vi "PH_ImageCoG_Plotter.Show Data.vi"(0 "i ref in":refnum<vi>, 5 "error in":errorcluster) -> (14 "i ref out":refnum<vi>, 19 "error out":errorcluster)   [LabVIEW 2014, in "PH_ImageCoG_Plotter.lvlib"]
doc: "This VI plots the data at the GUI elements."
uses:
  PH_ImageCoG_Plotter.lvlib
  <vilib>/Analysis/NI_AALBase.lvlib
  <vilib>/Analysis/NI_AALPro.lvlib
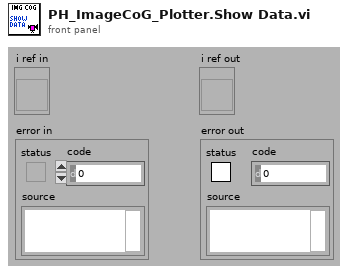
[diagram p1: front panel]
types:
  T1 = typedef "PH_ImageCoG_Plotter.lvlib/PH_ImageCoG_Plotter.i attribute.ctl" = cluster{"GUI Refs":cluster{"Delete":refnum<vi>, "Calibration status":refnum<vi>, "BI subtracted":refnum<vi>, "calc Beam Anal":refnum<vi>, "CoG - x":refnum<vi>, "CoG - y":refnum<vi>, "Type":refnum<vi>, "Center":refnum<vi>, "exp - X":refnum<vi>, "exp - Y":refnum<vi>, "Delta - X":refnum<vi>, "Delta - Y":refnum<vi>, "Available Cams":refnum<vi>, "CoG X":refnum<vi>, "CoG Y":refnum<vi>, "Delta X":refnum<vi>, "Delta Y":refnum<vi>, "Export Data":refnum<vi>, "Calibration data":refnum<vi>}, "Calibration":cluster{"Status":T2, "Calibration data":T3, "Calibration Data File":path}, "Beam Analysis":cluster{"on":bool, "exp - X":i32, "exp - Y":i32, "Type":bool, "Data":cluster{"current time":timestamp, "CoG-x":dbl, "CoG-y":dbl, "Delta-x":dbl, "Delta-y":dbl}[], "Datasets strored":i32, "Dataarray Size":i32}, "Cam instances":string[], "DIM Service Events":T4[], "Images":cluster{"Background":T7, "OP":T7, "GUI":T7}}
  T2 = typedef "PH_StatusHandler.lvlib/PH_StatusHandler.Status.ctl" = i16
  T3 = typedef "PH_ImageCalibrator.lvlib/PH_ImageCalibrator.Calibration Data.ctl" = cluster{"Date":string, "Time":string, "Cam Settings":cluster{"Cam ID":string, "Gain":dbl, "Brightness":dbl, "Shutter":dbl, "Cam Error":bool, "Mode":i32}, "Background Image":cluster{"Image":dbl[][], "Image Error":bool}, "Linear Calibration":cluster{"Calibration Factor":dbl, "not mm or mrad":bool}, "Energy Calibration":cluster{"Calibration Factor":dbl, "no mJ":bool}}
  T4 = typedef "BaseProcess.lvlib/BaseProcess.event definition.ctl" = cluster{"CAEEvtDef":T5, "Data Descriptor":T6}
  T5 = typedef "CAEObj.lvlib/CAEObj.event definition.ctl" = cluster{"URL":string, "enable":bool, "ignoreResID":bool}
  T6 = typedef "BaseProcess.lvlib/BaseProcess.descriptor string definition.ctl" = string
  T7 = typedef "IMAQ Image.ctl" = refnum<image>
  T8 = cluster{"current time":timestamp, "CoG-x":dbl, "CoG-y":dbl, "Delta-x":dbl, "Delta-y":dbl}[]
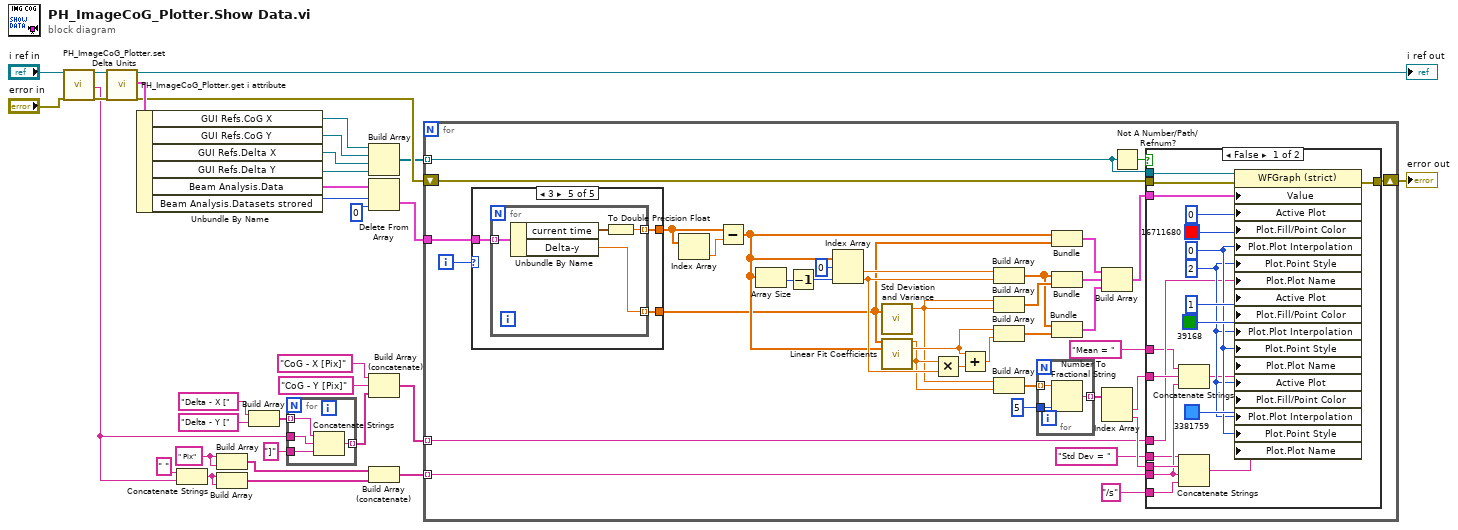
[diagram p0: block diagram]
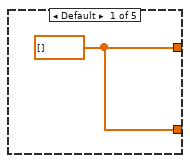
[diagram p2: hidden frame]
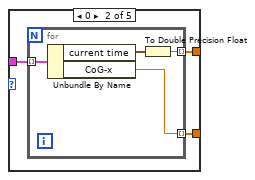
[diagram p3: hidden frame]
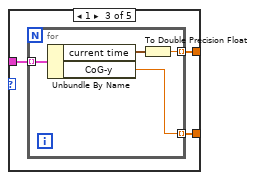
[diagram p4: hidden frame]
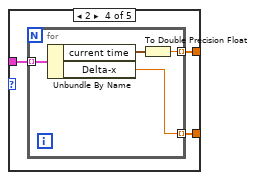
[diagram p5: hidden frame]
diagram:
  w12 = " Pix" ("Plot.Plot Name")
  n1 = call "PH_ImageCoG_Plotter.set Delta Units.vi"("i ref in"="i ref in", "error in (no error)"="error in") -> ("i ref out"=w24:refnum<vi>, "Unit"=w5:string, "error out"=w22:errorcluster)  [unwired: 15 in]
  n2 = call "PH_ImageCoG_Plotter.get i attribute.vi"("i ref in"=w24, "error in (no error)"=w22) -> ("i ref out"=→"i ref out":refnum<vi>, "i attribute"=w32:T1, "error out"=w27:errorcluster)  [unwired: 15 in]
  n3 = Unbundle By Name(w32) -> ("GUI Refs.CoG X"=w9:refnum<vi>, "GUI Refs.CoG Y"=w17:refnum<vi>, "GUI Refs.Delta X"=w16:refnum<vi>, "GUI Refs.Delta Y"=w15:refnum<vi>, "Beam Analysis.Data"=w4:T8, "Beam Analysis.Datasets strored"=w3:i32)
  n4 = Concatenate Strings(" " ("string"), w5) -> (w7:string)
  n5 = Build Array(w12, w12) -> (w13:string[])
  n6 = Build Array(w7, w7) -> (w14:string[])
  n7 = Build Array("Delta - X [" ("Plot.Plot Name"), "Delta - Y [" ("Plot.Plot Name")) -> (w18:string[])
  n8 = for {
    tunnel: w18 -> [w36] mode=indexing
    tunnel: "]" ("Plot.Plot Name") -> [w35]
    tunnel: w5 -> [w34]
    tunnel: [w33] -> w21 mode=indexing
    n9 = Concatenate Strings(w36, w34, w35) -> (w33:string)
  }
  n10 = Build Array(w9, w17, w16, w15) -> (w8:refnum<vi>[])
  n11 = Delete From Array(array=w4, length=w3, index=0) -> (deleted portion=w1:T8)  [unwired: 1 out]
  n12 = Build Array (concatenate)("CoG - X [Pix]" ("Plot.Plot Name"), "CoG - Y [Pix]" ("Plot.Plot Name"), w21) -> (w10:string[])
  n13 = Build Array (concatenate)(w13, w14) -> (w11:string[])
  n14 = for {
    tunnel: w8 -> [w70] mode=indexing
    tunnel: w11 -> [w69] mode=indexing
    shift-right: [w73] -> w31
    shift-left: w27 -> [w71]
    tunnel: w10 -> [w46] mode=indexing
    tunnel: w1 -> [w40]
    i -> [w37]
    n15 = case shown="3" w37 {
      tunnel: [w74 w77 w84 w91 w98] -> w41
      tunnel: w40 -> [_ w76 w83 w90 w97]
      tunnel: [w74 w75 w82 w89 w96] -> w38
      frame Default {
        w74 = dbl[] []
      }
      frame 0 {
        n16 = for {
          tunnel: w76 -> [w81] mode=indexing
          tunnel: [w78] -> w77 mode=indexing
          tunnel: [w80] -> w75 mode=indexing
          n17 = Unbundle By Name(w81) -> ("current time"=w79:timestamp, "CoG-x"=w80:dbl)
          n18 = To Double Precision Float(number=w79) -> (double precision float=w78:dbl)
        }
      }
      frame 1 {
        n19 = for {
          tunnel: w83 -> [w88] mode=indexing
          tunnel: [w85] -> w84 mode=indexing
          tunnel: [w87] -> w82 mode=indexing
          n20 = Unbundle By Name(w88) -> ("current time"=w86:timestamp, "CoG-y"=w87:dbl)
          n21 = To Double Precision Float(number=w86) -> (double precision float=w85:dbl)
        }
      }
      frame 2 {
        n22 = for {
          tunnel: w90 -> [w95] mode=indexing
          tunnel: [w92] -> w91 mode=indexing
          tunnel: [w94] -> w89 mode=indexing
          n23 = Unbundle By Name(w95) -> ("current time"=w93:timestamp, "Delta-x"=w94:dbl)
          n24 = To Double Precision Float(number=w93) -> (double precision float=w92:dbl)
        }
      }
      frame 3 {
        n25 = for {
          tunnel: w97 -> [w102] mode=indexing
          tunnel: [w99] -> w98 mode=indexing
          tunnel: [w101] -> w96 mode=indexing
          n26 = Unbundle By Name(w102) -> ("current time"=w100:timestamp, "Delta-y"=w101:dbl)
          n27 = To Double Precision Float(number=w100) -> (double precision float=w99:dbl)
        }
      }
    }
    n28 = Index Array(array=w41) -> (element=w42:dbl)  [unwired: 1 in]
    n29 = Subtract(x=w41, y=w42) -> (x-y=w39:dbl[])
    n30 = Array Size(array=w39) -> (size(s)=w66:i32)
    n31 = Decrement(x=w66) -> (x-1=w65:i32)
    n32 = Index Array(array=w39, index #1=0 ("index"), index #2=w65) -> (element #1=w63:dbl, element #2=w55:dbl)
    n33 = call <vilib>:"Std Deviation and Variance.vi"("X"=w38) -> ("mean"=w53:dbl)  [unwired: 1 in, 2 out]
    n34 = call <vilib>:"Linear Fit Coefficients.vi"("Y"=w38, "X"=w39) -> ("slope"=w54:dbl, "intercept"=w58:dbl)  [unwired: 11 in, 1 out]
    n35 = Multiply(x=w54, y=w55) -> (x*y=w61:dbl)
    n36 = Add(x=w58, y=w61) -> (x+y=w57:dbl)
    n37 = Build Array(w63, w55) -> (w59:dbl[])
    n38 = Build Array(w53, w53) -> (w62:dbl[])
    n39 = Build Array(w58, w57) -> (w56:dbl[])
    n40 = Build Array(w53, w54) -> (w52:dbl[])
    n41 = for {
      tunnel: w52 -> [w105] mode=indexing
      tunnel: [w104] -> w51 mode=indexing
      tunnel: i16 5 ("precision (6)") -> [w103]
      n42 = Number To Fractional String(number=w105, precision (6)=w103) -> (F-format string=w104:string)  [unwired: 2 in]
    }
    n43 = Bundle(w39, w38) -> (w68:cluster{dbl[], dbl[]})  [unwired: 1 in]
    n44 = Bundle(w59, w62) -> (w67:cluster{dbl[], dbl[]})  [unwired: 1 in]
    n45 = Bundle(w59, w56) -> (w60:cluster{dbl[], dbl[]})  [unwired: 1 in]
    n46 = Build Array(w68, w67, w60) -> (w49:cluster{dbl[], dbl[]}[])
    n47 = Index Array(array=w51) -> (element #1=w48:string, element #2=w47:string)  [unwired: 2 in]
    n48 = Not A Number/Path/Refnum?(number/path/refnum=w70) -> (NaN/Path/Refnum?=w72:bool)
    n49 = case shown="False" w72 {
      tunnel: w70 -> [w120 _]
      tunnel: w71 -> [w122 w126]
      tunnel: [w121 w126] -> w73
      tunnel: w48 -> [w113 _]
      tunnel: w47 -> [w114 _]
      tunnel: w69 -> [w112 _]
      tunnel: w46 -> [w111 _]
      tunnel: w49 -> [w109 _]
      tunnel: "Std Dev = " ("Plot.Plot Name") -> [w108 _]
      tunnel: "Mean = " ("Plot.Plot Name") -> [w107 _]
      tunnel: "/s" ("Plot.Plot Name") -> [w106 _]
      frame False {
        w118 = u8 0 ("Plot.Plot Interpolation")
        w117 = u8 2 ("Plot.Plot Interpolation")
        n50 = Concatenate Strings(w107, w113, w112) -> (w116:string)
        n51 = Concatenate Strings(w108, w114, w112, w106) -> (w115:string)
        n52 = property class="WFGraph (strict)"(reference=w120, error in=w122, "Value"=w109, "Active Plot"=u32 0, "Plot.Fill/Point Color"=u32 16711680 ("Color Box"), "Plot.Plot Interpolation"=w118, "Plot.Point Style"=w117, "Plot.Plot Name"=w111, "Active Plot"=u32 1, "Plot.Fill/Point Color"=u32 39168 ("Color Box"), "Plot.Plot Interpolation"=w117, "Plot.Point Style"=w118, "Plot.Plot Name"=w116, "Active Plot"=w117, "Plot.Fill/Point Color"=u32 3381759 ("Color Box"), "Plot.Plot Interpolation"=w117, "Plot.Point Style"=w118, "Plot.Plot Name"=w115) -> (error out=w121:errorcluster)  [unwired: 1 out]
      }
      frame True {
      }
    }
  }
  "error out" <- w31
